vi "信息录入.vi"(2 "?":i32(ring) items=["0", "1", "2", "3", "4", "5", "6", "7", "8", "9", "10", "11", "12", "13", "14", "15", "16", "17", "18", "19", "20"]) -> (0 "年龄 2":u8, 1 "成员 2":string, 3 "表格控件":string[][](table))   [LabVIEW 2016]
uses:
  <vilib>/Utility/file.llb/Read Delimited Spreadsheet (string).vi
panel:
  # "成员选择"
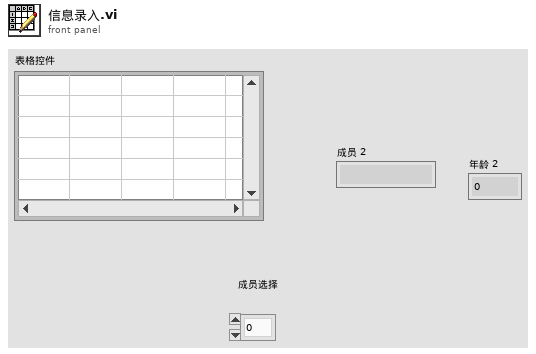
[diagram p1: front panel]
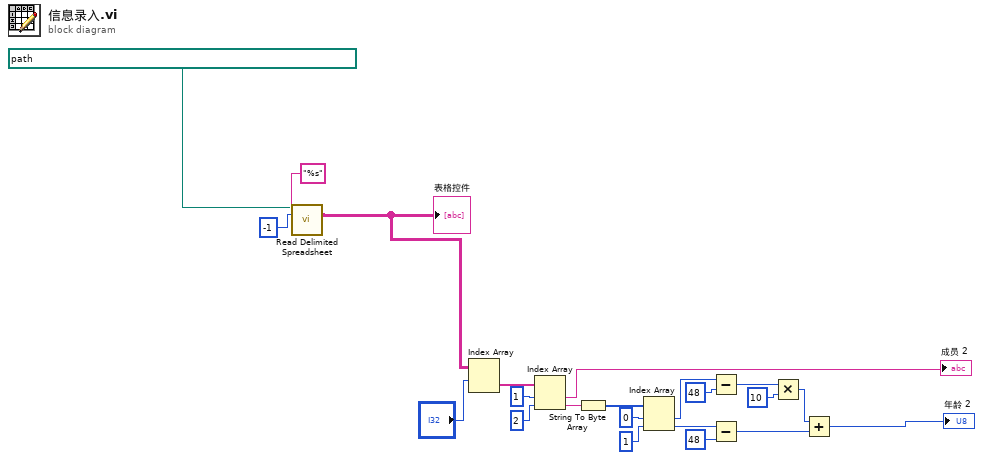
[diagram p0: block diagram]
diagram:
  n1 = call-poly <vilib>:"Read Delimited Spreadsheet.vi"("file path (dialog if empty)"=path "C:/Users/Administrator/Desktop/课程设计/家庭成员信息.txt" ("基路径"), "format (%s)"="%s" ("format (%d)"), "number of rows (all:-1)"=-1) -> ("all rows"=w2:string[][])  [unwired: 7 in, 5 out]
  "表格控件" <- w2
  n2 = Index Array(array=w2, index (row)="?") -> (element=w21:string[])  [unwired: 1 in]
  n3 = Index Array(array=w21, index #1=1 ("索引"), index #2=2 ("索引")) -> (element #1=→"成员 2":string, element #2=w18:string)
  n4 = String To Byte Array(string=w18) -> (unsigned byte array=w17:u8[])
  n5 = Index Array(array=w17, index #1=0 ("索引"), index #2=1 ("索引")) -> (element #1=w15:u8, element #2=w14:u8)
  n6 = Subtract(x=w15, y=u8 48) -> (x-y=w12:u8)
  n7 = Subtract(x=w14, y=u8 48) -> (x-y=w9:u8)
  n8 = Multiply(x=w12, y=u8 10) -> (x*y=w10:u8)
  n9 = Add(x=w10, y=w9) -> (x+y=→"年龄 2":u8)
